vi "Read (DBL with Units).vi"(6 "ISOBUS address":T3=-1 caption="ISOBUS address (-1)", 8 "error in":errorcluster, 10 "SCPI Message(s)":string[](array[string]), 11 "Mercury Reference In":T4) -> (0 "error out":errorcluster, 1 "Unit":T1, 2 "Data (Dbl)":dbl, 3 "Mercury Reference Out":T4, 4 "Valid?":T2)   [LabVIEW 2019, in "Mercury iXX.lvlib"]
doc: "Read the response from the instrument and outputs the result as a numeric with a unit response as a string indicator."
uses:
  Mercury iXX.lvlib
  Public/Controls/Mercury Reference.ctl
  Public/Controls/Comms Transport Layer.ctl
  Controls/Query Dynamic Reference.ctl
  Public/Controls/ISOBus Address.ctl
  Public/Controls/Is Valid LED.ctl
  Public/Controls/Unit String.ctl
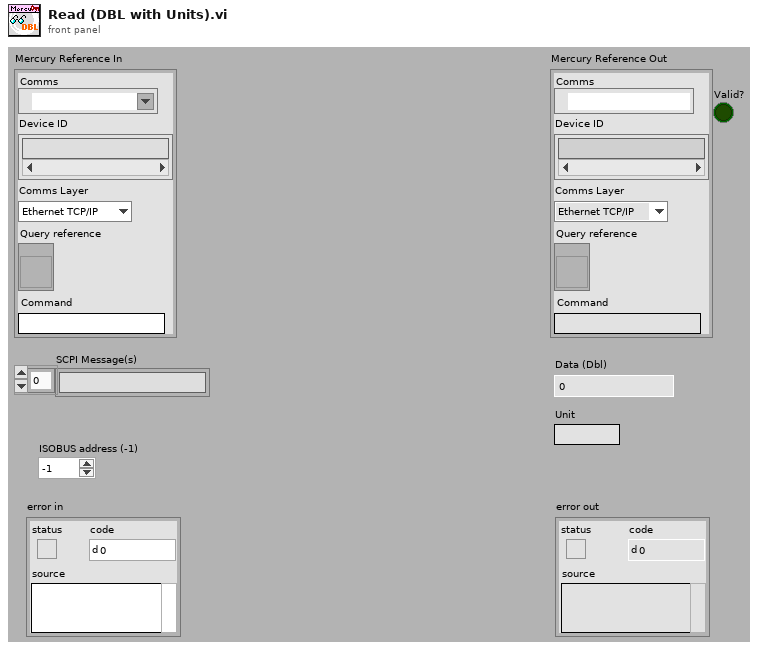
[diagram p1: front panel]
types:
  T1 = typedef "Mercury iXX.lvlib/Unit String.ctl" = string
  T2 = typedef "Mercury iXX.lvlib/Is Valid LED.ctl" = bool
  T3 = typedef "Mercury iXX.lvlib/ISOBus Address.ctl" = i32
  T4 = typedef "Mercury iXX.lvlib/Mercury Reference.ctl" = cluster{"Comms":refnum<visa-resource-name>, "Device ID":string[], "Comms Layer":T5, "Command":string, "Query reference":T6}
  T5 = typedef "Mercury iXX.lvlib/Comms Transport Layer.ctl" = enum16{"Ethernet TCP/IP", "USB", "ISOBus - RS-232", "GPIB"}
  T6 = typedef "Mercury iXX.lvlib/Query Dynamic Reference.ctl" = refnum<vi>
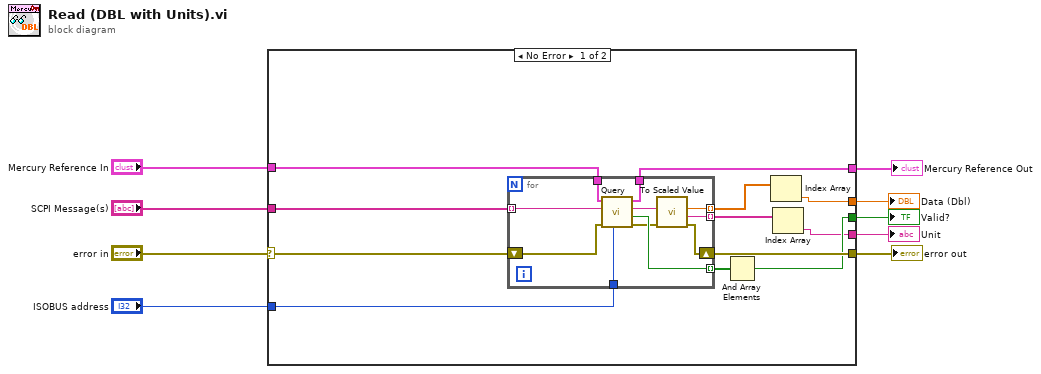
[diagram p0: block diagram]
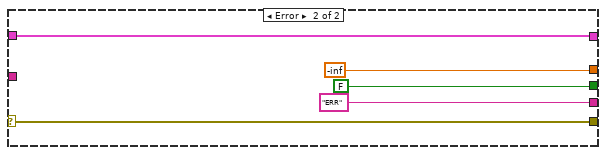
[diagram p2: hidden frame]
diagram:
  n1 = case shown="No Error" "error in" {
    selector: "error in" -> [w19 w36]
    tunnel: "Mercury Reference In" -> [w17 w37]
    tunnel: [w16 w37] -> w8
    tunnel: [w15 w36] -> w7
    tunnel: "ISOBUS address" -> [w18 _]
    tunnel: [w11 -inf] -> w4
    tunnel: [w14 FALSE ("Valid?")] -> w3
    tunnel: [w12 "ERR" ("Unit")] -> w2
    tunnel: "SCPI Message(s)" -> [w10 _]
    frame No Error {
      n2 = for {
        tunnel: [w26] -> w20 mode=indexing
        tunnel: w17 -> [w32]
        shift-right: [w23] -> w15
        shift-left: w19 -> [w31]
        tunnel: [w30] -> w21 mode=indexing
        tunnel: w18 -> [w29]
        tunnel: [w28] -> w16
        tunnel: [w25] -> w13 mode=indexing
        tunnel: w10 -> [w22] mode=indexing
        n3 = call "Query.vi"("ISOBUS address"=w29, "error in"=w31, "Command"=w22, "Mercury Reference In"=w32) -> ("error out"=w24:errorcluster, "Valid?"=w30:bool, "Data"=w27:string, "Mercury Reference Out"=w28:T4)  [unwired: 1 in, 3 out]
        n4 = call "To Scaled Value.vi"("error in"=w24, "Response"=w27) -> ("error out"=w23:errorcluster, "Unit"=w25:T1, "Scaled Value"=w26:dbl)  [unwired: 7 out]
      }
      n5 = And Array Elements(Boolean array=w21) -> (logical AND=w14:bool)
      n6 = Index Array(array=w20) -> (element=w11:dbl)  [unwired: 1 in]
      n7 = Index Array(array=w13) -> (element=w12:T1)  [unwired: 1 in]
    }
    frame Error {
    }
  }
  "Mercury Reference Out" <- w8
  "error out" <- w7
  "Data (Dbl)" <- w4
  "Valid?" <- w3
  "Unit" <- w2
